vi "CollectAsyncMessageResponseCore.vi"(8 "error in (no error)":errorcluster, 10 "Wait for All Messages?":bool, 11 "MicronGRPCClient in":refnum<class "MicronGRPCClient.lvclass">) -> (0 "error out":errorcluster, 2 "Responses":T1[](array[typedef]), 3 "MicronGRPCClient out":refnum<class "MicronGRPCClient.lvclass">)   [LabVIEW 2019, in "MicronGRPCClient.lvclass"]
uses:
  MicronGRPCClient.lvclass
  Typedefs/AsyncMessageResponse.ctl
  Generated/MicronGRPCGeneratedClient/RPC Messages/micronGrpc_MessageRequest.ctl
  MicronGRPCClient.lvclass/MicronGRPCClient.ctl
  31872622-b810-4eaf-963a-5b51371864dd.vi
  Generated/MicronGRPCGeneratedClient/MicronGRPCGeneratedClient.lvlib
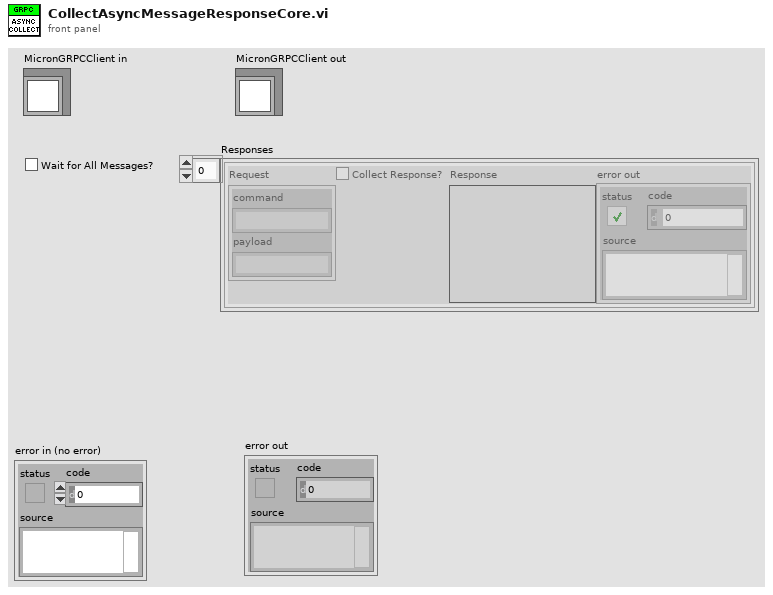
[diagram p1: front panel]
types:
  T1 = typedef "MicronGRPCClient.lvclass/AsyncMessageResponse.ctl" = cluster{"Request":T2, "Collect Response?":bool, "Response":string, "error out":errorcluster}
  T2 = typedef "MicronGRPCGeneratedClient.lvlib/micronGrpc_MessageRequest.ctl" = cluster{"command":string, "payload":string}
  T3 = typedef "MicronGRPCClient.lvclass/AsyncCluster.ctl" = cluster{"InputQueue":refnum<queue>, "OutputQueue":refnum<queue>}
  T4 = typedef "SLL QSM.lvlib/Queue Type.ctl" = cluster{"State":string, "Data":variant}
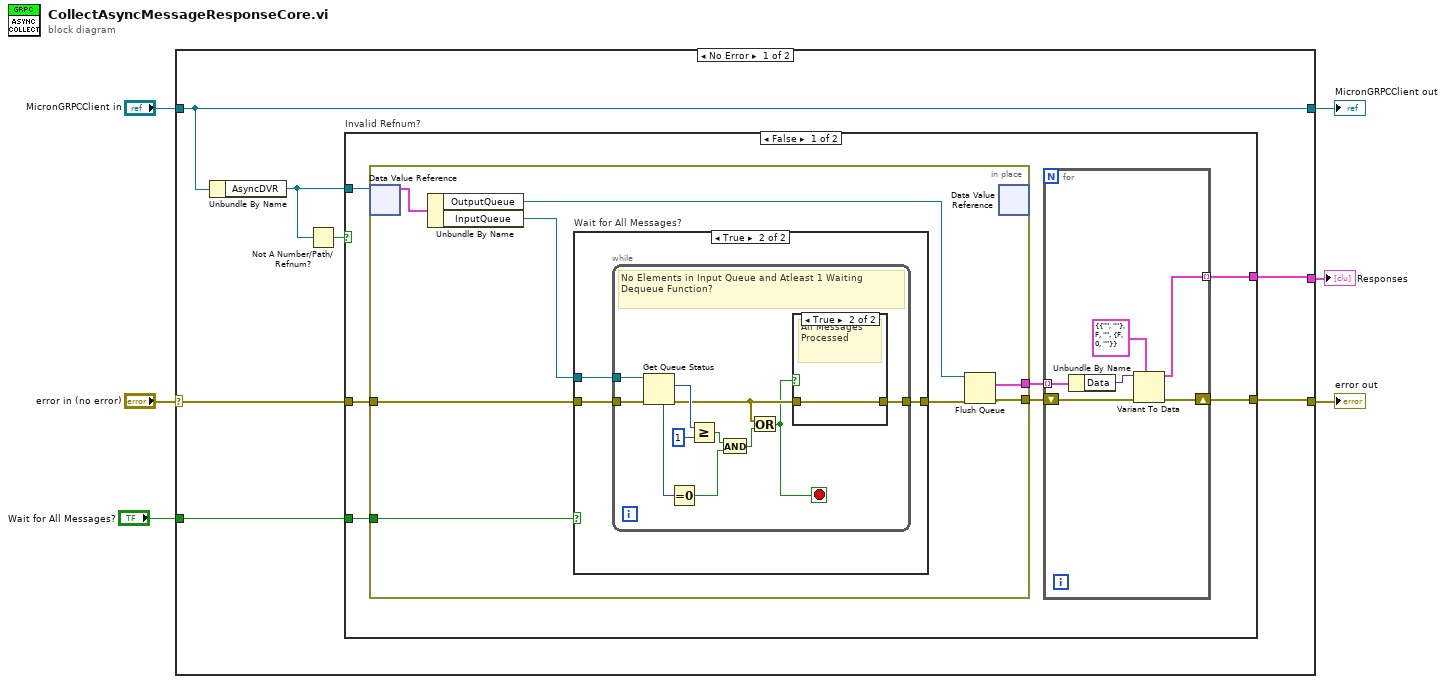
[diagram p0: block diagram]
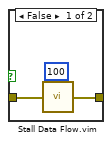
[diagram p3: hidden frame]
diagram:
  n1 = case shown="No Error" "error in (no error)" {
    selector: "error in (no error)" -> [w12 w56]
    tunnel: [w11 w56] -> w5
    tunnel: [w13 w55] -> w3
    tunnel: "MicronGRPCClient in" -> [w13 w55]
    tunnel: [w10 _] -> w2
    tunnel: "Wait for All Messages?" -> [w9 _]
    frame No Error {
      n2 = Unbundle By Name(w13) -> ("AsyncDVR"=w8:refnum<data-value>)
      n3 = Not A Number/Path/Refnum?(number/path/refnum=w8) -> (NaN/Path/Refnum?=w7:bool)
      n4 = case "Invalid Refnum?" shown="False" w7 {
        tunnel: w12 -> [w20 w54]
        tunnel: [w19 w54] -> w11
        tunnel: [w18 _] -> w10
        tunnel: w9 -> [w17 _]
        tunnel: w8 -> [w14 _]
        frame False {
          n5 = in-place {
            in-place-border: w20 -> [w30]
            in-place-border: [w32] -> w16
            in-place-border: [w31] -> w15
            in-place-border: w17 -> [w27]
            n6 = in-place-dvr #1(w14) -> (w34:T3)  [unwired: 1 out]
            n7 = Unbundle By Name(w34) -> ("OutputQueue"=w33:refnum<queue>, "InputQueue"=w28:refnum<queue>)
            n8 = case "Wait for All Messages?" shown="True" w27 {
              tunnel: w30 -> [w35 w38]
              tunnel: [w35 w37] -> w29
              tunnel: w28 -> [_ w36]
              frame False {
              }
              frame True {
                n9 = while {
                  tunnel: w38 -> [w49]
                  tunnel: [w46] -> w37
                  tunnel: w36 -> [w48]
                  stop <- w39 stop-if-true
                  # "No Elements in Input Queue and Atleast 1 Waiting Dequeue Function?"
                  n10 = Get Queue Status(queue=w48, error in (no error)=w49) -> (# pending remove=w45:i32, error out=w40:errorcluster, # elements in queue=w47:i32)  [unwired: 1 in, 5 out]
                  n11 = Equal To 0?(x=w47) -> (x = 0?=w42:bool)
                  n12 = Greater Or Equal?(x=w45, y=1) -> (x >= y?=w43:bool)
                  n13 = And(x=w43, y=w42) -> (x .and. y?=w41:bool)
                  n14 = Or(x=w40, y=w41) -> (x .or. y?=w39:bool)
                  n15 = case shown="True" w39 {
                    tunnel: w40 -> [w52 w53]
                    tunnel: [w51 w53] -> w46
                    frame False {
                      n16 = call "Stall Data Flow.vim"("value in"=w52, "milliseconds to wait"=u32 100) -> ("value out"=w51:errorcluster)  [unwired: 1 out]
                    }
                    frame True {
                      # "All Messages Processed"
                    }
                  }
                }
              }
            }
            n17 = Flush Queue(queue=w33, error in (no error)=w29) -> (remaining elements=w31:T4[], error out=w32:errorcluster)  [unwired: 1 out]
            n18 = in-place-dvr #1() -> ()  [unwired: 1 in, 2 out]
          }
          n19 = for {
            shift-right: [w25] -> w19
            shift-left: w16 -> [w26]
            tunnel: w15 -> [w24] mode=indexing
            tunnel: [w21] -> w18 mode=indexing
            n20 = Unbundle By Name(w24) -> ("Data"=w23:variant)
            n21 = Variant To Data(error in=w26, type=T1 {"Request"={"command"="", "payload"=""}, "Collect Response?"=FALSE, "Response"="", "error out"={"status"=FALSE, "code"=0, "source"=""}} ("AsyncResponse"), Variant=w23) -> (data=w21:T1, error out=w25:errorcluster)
          }
        }
        frame True {
        }
      }
    }
    frame Error {
    }
  }
  "error out" <- w5
  "MicronGRPCClient out" <- w3
  "Responses" <- w2
